vi "setData.vi"(8 "error in (no error)":errorcluster, 10 "Data":string[][](array[string]), 11 "reference in":refnum<class "PartsTracking Controller.lvclass">) -> (0 "error out":errorcluster, 3 "reference out":refnum<class "PartsTracking Controller.lvclass">)   [LabVIEW 2014, in "PartsTracking Controller.lvclass"]
uses:
  PartsTracking Controller.lvclass
  APP/excelFile_class/fileType.ctl
  File Controller_llb/File Controller.lvclass
  APP/excelFile_class/excelFile.lvclass
  APP/partsTracking_class/partsTracking.lvclass
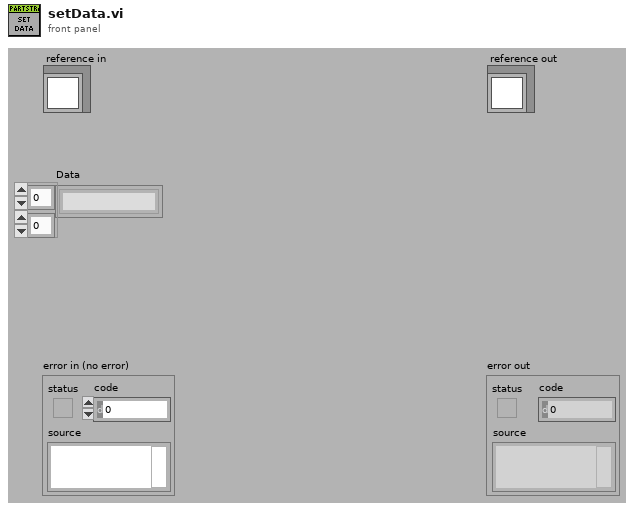
[diagram p1: front panel]
types:
  T1 = typedef "excelFile.lvclass/fileType.ctl" = enum16{"devices", "items", "partsTracking"}
  T2 = typedef "PartsTracking Controller.lvclass/ObjectAttributesRef.ctl" = refnum<data-value>
  T3 = typedef "PartsTracking Controller.lvclass/ObjectAttributes.ctl" = cluster{"MyAttribute":dbl, "file_controller_ref":refnum<class "File Controller.lvclass">, "data":string[][], "partsTracking_ref":refnum<class "partsTracking.lvclass">, "project_panels_ref":refnum<class "Project Panels.lvclass">}
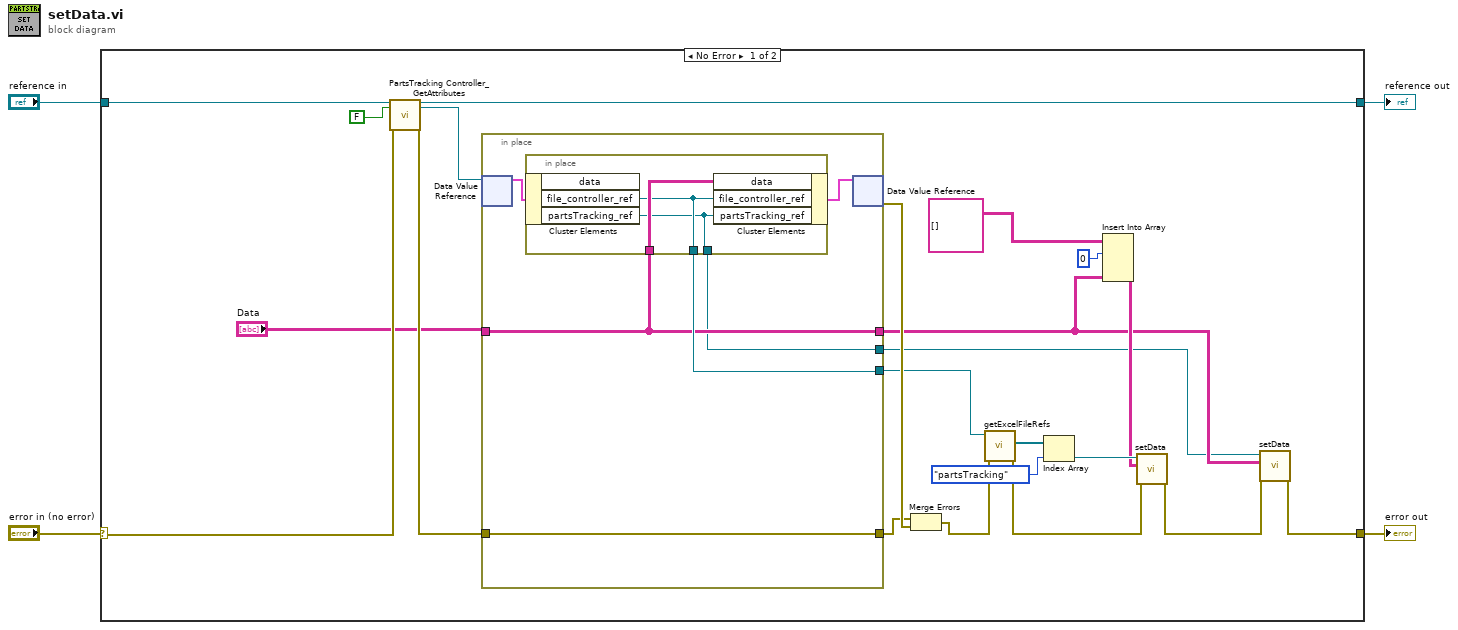
[diagram p0: block diagram]
diagram:
  n1 = case shown="No Error" "error in (no error)" {
    selector: "error in (no error)" -> [w22 w37]
    tunnel: [w7 w37] -> w3
    tunnel: [w20 w36] -> w1
    tunnel: "reference in" -> [w24 w36]
    frame No Error {
      n2 = call "PartsTracking Controller_GetAttributes.vi"("reference in"=w24, "return data? (T)"=FALSE, "error in (no error)"=w22) -> ("reference out"=w20:refnum<class "PartsTracking Controller.lvclass">, "attributes ref"=w19:T2, "error out"=w21:errorcluster)  [unwired: 13 in, 1 out]
      n3 = in-place {
        in-place-border: w21 -> [w30]
        in-place-border: [w30] -> w25
        in-place-border: "Data" -> [w28]
        in-place-border: [w29] -> w18
        in-place-border: [w28] -> w6
        in-place-border: [w27] -> w5
        n4 = in-place-dvr #1(w19) -> (w31:T3)  [unwired: 1 out]
        n5 = in-place {
          in-place-border: w28 -> [w35]
          in-place-border: [w34] -> w29
          in-place-border: [w33] -> w27
          n6 = in-place-cluster #2(w31) -> ("file_controller_ref"=w34:refnum<class "File Controller.lvclass">, "partsTracking_ref"=w33:refnum<class "partsTracking.lvclass">)  [unwired: 1 out]
          n7 = in-place-cluster #2("data"=w35, "file_controller_ref"=w34, "partsTracking_ref"=w33) -> (w32:T3)
        }
        n8 = in-place-dvr #1(w32) -> (w26:errorcluster)  [unwired: 1 out]
      }
      n9 = Merge Errors(w25, w26) -> (w17:errorcluster)
      n10 = call "getExcelFileRefs.vi"("error in (no error)"=w17, "reference in"=w18) -> ("error out"=w16:errorcluster, "excelFile_refs"=w15:refnum<class "excelFile.lvclass">[])  [unwired: 7 in, 1 out]
      n11 = Index Array(array=w15, index=fileType."partsTracking" ("fileType")) -> (element=w14:refnum<class "excelFile.lvclass">)
      n12 = Insert Into Array(array=string[][][] [] ("data"), index (dim 0)=0 ("disabled index (page)"), new element=w6) -> (w10:string[][][])  [unwired: 2 in]
      n13 = call "setData.vi"("error in (no error)"=w16, "data"=w10, "reference in"=w14) -> ("error out"=w8:errorcluster)  [unwired: 7 in, 1 out]
      n14 = call "setData.vi"("error in (no error)"=w8, "data"=w6, "reference in"=w5) -> ("error out"=w7:errorcluster)  [unwired: 7 in, 1 out]
    }
    frame Error {
    }
  }
  "error out" <- w3
  "reference out" <- w1
